vi "Create Path with Appended Integer.vi"(8 "error in (no error)":errorcluster, 10 "Path Number":u32, 11 "Base Path (in)":path) -> (0 "error out":errorcluster, 2 "Numeric Appended Path":path, 3 "Base Path (out)":path)   [LabVIEW 2016]
uses:
  <userlib>/_OpenG.lib/file/file.llb/Strip Path Extension - Path__ogtk.vi
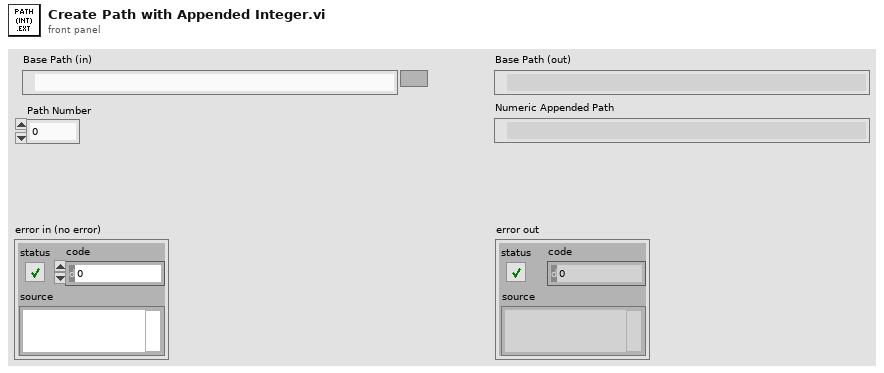
[diagram p1: front panel]
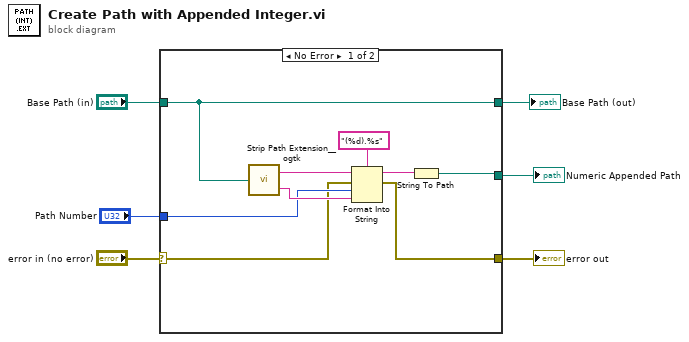
[diagram p0: block diagram]
diagram:
  n1 = case shown="No Error" "error in (no error)" {
    selector: "error in (no error)" -> [w10 w16]
    tunnel: "Base Path (in)" -> [w15 w17]
    tunnel: [w15 w17] -> w4
    tunnel: [w7 w16] -> w3
    tunnel: [w8 _] -> w2
    tunnel: "Path Number" -> [w12 _]
    frame No Error {
      n2 = call-poly <userlib>:"Strip Path Extension__ogtk.vi"("path"=w15) -> ("root"=w14:string, "extension"=w13:string)
      n3 = Format Into String(format string="(%d).%s", initial string=w14, error in=w10, w12, w13) -> (resulting string=w9:string, error out=w7:errorcluster)
      n4 = String To Path(string=w9) -> (path=w8:path)
    }
    frame Error {
    }
  }
  "Base Path (out)" <- w4
  "Numeric Appended Path" <- w2
  "error out" <- w3
